vi "STPDegub.vi"(0 "object in":refnum<class "Game.lvclass">, 5 "error in (no error)":errorcluster) -> (14 "object out":refnum<class "Game.lvclass">, 19 "error out":errorcluster)   [LabVIEW 2023, in "Game.lvclass"]
uses:
  Game.lvclass
  Zone_class/zones.ctl
  Zone_class/Zone.lvclass
  Robot_class/roles.ctl
  Game.lvclass/Game.ctl
  Team_class/Team.lvclass/Team.ctl
  Field_class/Field.lvclass/Field.ctl
  PrimaryAttacker_class/PrimaryAttackerRole.lvclass
  C:/Users/ebert/Documents/codes/SSL/repo/SSL_AI/NewSTP/NewRoles/Role_v2_class/Role_v2.lvclass
  SupportAttackerRole/SupportAttackerRole.lvclass
  SupportAttackerRole/SupportAttackerRole_states.ctl
  PrimaryAttacker_class/PrimaryAttackerRole_states.ctl
  Robot_class/Robot.lvclass/Robot.ctl
  Robot_class/Write role.vi
  Read AllyRef.vi
  Read FieldRef.vi
  Field_class/Read enemyGoalPosition.vi
  Team_class/Read RobotRef.vi
  Read OffensiveTeam.vi
  Team_class/Write RobotRef.vi
  Write OffensiveTeam.vi
  Ally_class/Ally.lvclass
  C:/Users/ebert/Documents/codes/SSL/repo/SSL_AI/Team_class/Team.lvclass
  NewSTP/Playbook_v2_class/Playbook_v2.lvclass
  Field_class/Field.lvclass
  Robot_class/Robot.lvclass
  NewSTP/NewPlays/Play_v2_class/Play_v2.lvclass
  ShootTactic_v2_class/ShootTactic_v2.lvclass
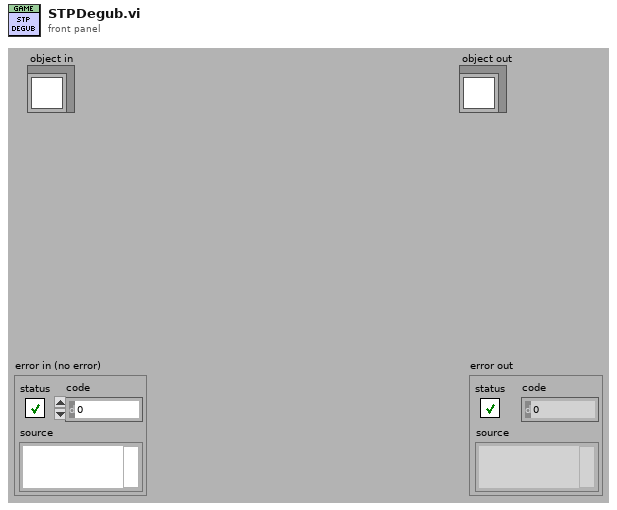
[diagram p1: front panel]
types:
  T1 = typedef "roles.ctl" = enum16{"SimpleBallPlacement", "BallPlacementAllyPasser", "BallPlacementAllyReceiver", "BallPlacementEnemy", "5Robots5th", "PassBestReceiver", "5Robots4th", "5Robots3rd", "5Robots2nd", "5Robots1st", "PassBestRobot", "WaitPass", "ABCThirdKicker", "ABCFirstKicker", "ABCSecondKicker", "Tabler", "TableFinalizer", "PrepareRollToPassRoller", "PrepareRollToPassReceiver", "SimplePassRoll", "SimplePassRollReceiver", "PenaltyDefense", "PreparePassReceiver 2", "PreparePassReceiver 1", "PassObserver", "Timeout", "Goto", "ZigZag", "None", "BallOutOfField", "DefenderArea", "Duelist", "AttackerStop", "FollowAttacker", "KeeperRole", "KickPenalty", "AttackerAimGoal", "AttackerBlock", "Marker", "Halt", "Shoot", "PassKicker", "PassReceiver", "TestRole", "PenaltyAttacker", "PrimaryAttackerRole", "SupportAttackerRole"}
  T2 = typedef "Zone.lvclass/zones.ctl" = enum16{"leftMidField", "rightMidField", "MidField", "leftWing", "rightWing", "LeftSide", "RightSide", "Field", "Size"}
  T3 = typedef "PrimaryAttackerRole.lvclass/PrimaryAttackerRole_states.ctl" = enum16{"Intercept", "PrepareShot", "Shoot", "Pass"}
  T4 = typedef "SupportAttackerRole.lvclass/SupportAttackerRole_states.ctl" = enum16{"Position", "WaitPass", "Exit"}
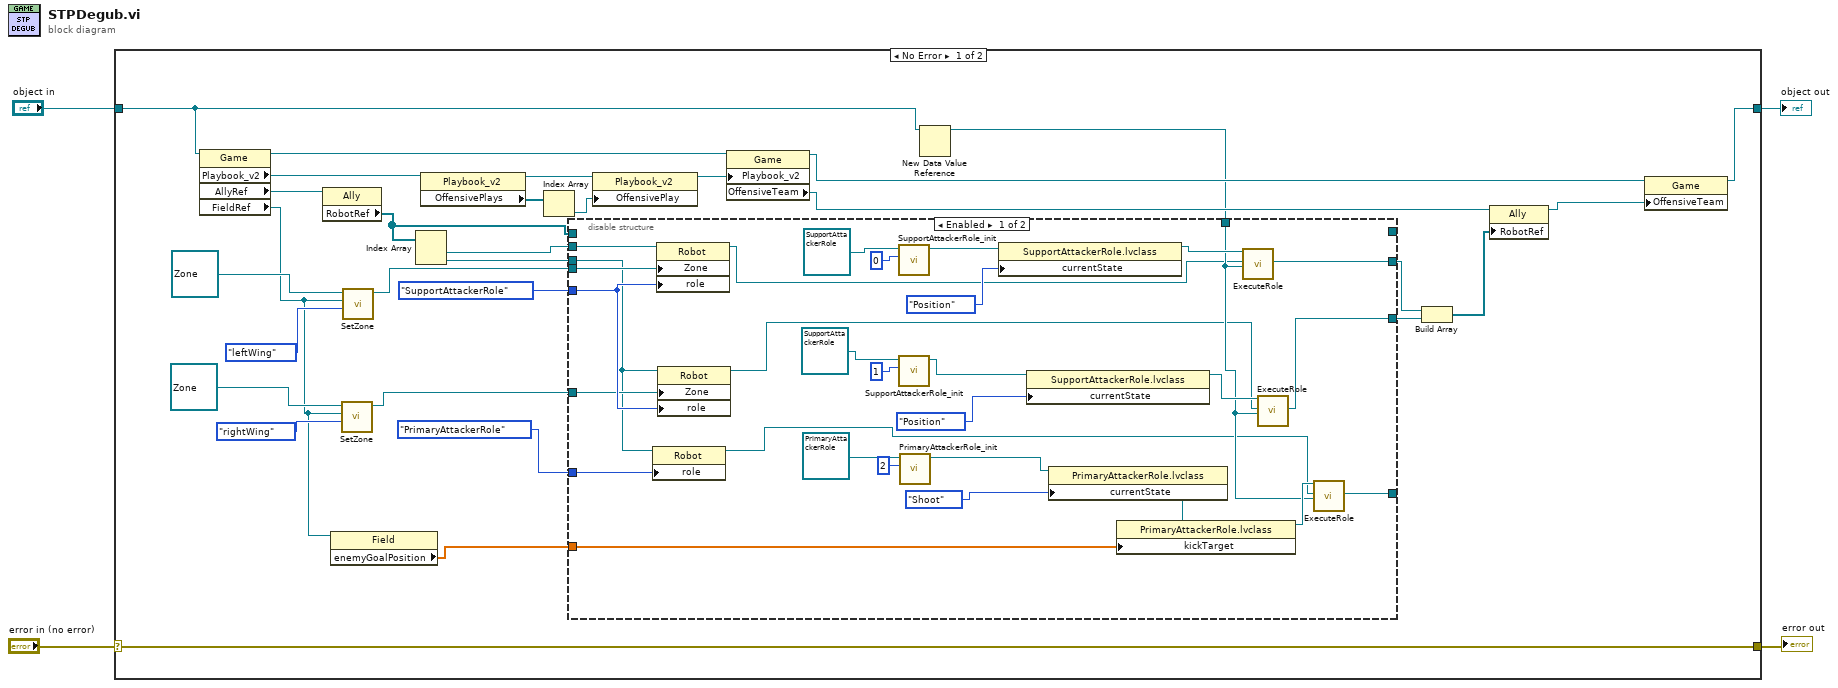
[diagram p0: block diagram]
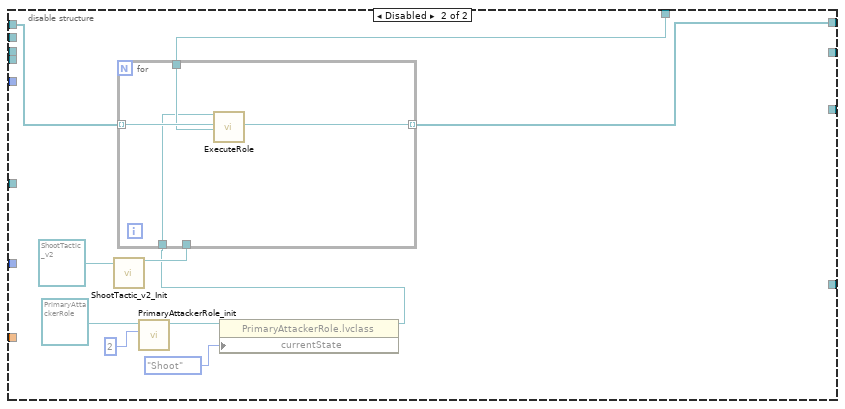
[diagram p2: hidden frame]
diagram:
  n1 = case shown="No Error" "error in (no error)" {
    selector: "error in (no error)" -> [w34 w80]
    tunnel: [w34 w80] -> w3
    tunnel: [w14 w79] -> w1
    tunnel: "object in" -> [w15 w79]
    frame No Error {
      n2 = property class="Game"(reference=w15) -> (reference out=w20:refnum<class "Game.lvclass">, "Playbook_v2"=w33:refnum<class "Playbook_v2.lvclass">, "AllyRef"=w29:refnum<class "Ally.lvclass">, "FieldRef"=w13:refnum<class "Field.lvclass">)  [unwired: 1 in, 1 out]
      n3 = property class="Ally"(reference=w29) -> ("RobotRef"=w8:refnum<class "Robot.lvclass">[])  [unwired: 1 in, 2 out]
      n4 = property class="Field"(reference=w13) -> ("enemyGoalPosition"=w12:dbl[])  [unwired: 1 in, 2 out]
      n5 = call-dynamic "SetZone.vi"("Enum"=zones."rightWing", "Field"=w13, "object in"=refnum<class "Zone.lvclass"> refnum ("Zone")) -> ("object out"=w24:refnum<class "Zone.lvclass">)  [unwired: 7 in, 1 out]
      n6 = call-dynamic "SetZone.vi"("Enum"=zones."leftWing", "Field"=w13, "object in"=refnum<class "Zone.lvclass"> refnum ("Zone")) -> ("object out"=w22:refnum<class "Zone.lvclass">)  [unwired: 7 in, 1 out]
      n7 = Index Array(array=w8) -> (element #1=w10:refnum<class "Robot.lvclass">, element #2=w9:refnum<class "Robot.lvclass">)  [unwired: 2 in]
      n8 = property class="Playbook_v2"(reference=w33) -> (reference out=w31:refnum<class "Playbook_v2.lvclass">, "OffensivePlays"=w32:refnum<class "Play_v2.lvclass">[])  [unwired: 1 in, 1 out]
      n9 = Index Array(array=w32) -> (element=w30:refnum<class "Play_v2.lvclass">)  [unwired: 1 in]
      n10 = property class="Playbook_v2"(reference=w31, "OffensivePlay"=w30) -> (reference out=w19:refnum<class "Playbook_v2.lvclass">)  [unwired: 1 in, 1 out]
      n11 = property class="Game"(reference=w20, "Playbook_v2"=w19) -> (reference out=w16:refnum<class "Game.lvclass">, "OffensiveTeam"=w17:refnum<class "Ally.lvclass">)  [unwired: 1 in, 1 out]
      n12 = New Data Value Reference(data value=w15) -> (data value reference=w11:refnum<data-value>)  [unwired: 1 in, 1 out]
      n13 = disable-structure shown="Enabled" {
        disable-tunnel: roles."SupportAttackerRole" ("role") -> [w64 _]
        disable-tunnel: w24 -> [w63 _]
        disable-tunnel: w22 -> [w62 _]
        disable-tunnel: roles."PrimaryAttackerRole" ("role") -> [w61 _]
        disable-tunnel: w12 -> [w45 _]
        disable-tunnel: w11 -> [w42 w66]
        disable-tunnel: w10 -> [w43 _]
        disable-tunnel: w9 -> [w35 _]
        disable-tunnel: [w41 _] -> _
        disable-tunnel: w8 -> [_ w74]
        disable-tunnel: [_ w65] -> _
        disable-tunnel: [w37 _] -> w7
        disable-tunnel: [w36 _] -> w6
        frame Enabled {
          n14 = property class="Robot"(reference=w35, "role"=w61) -> (reference out=w38:refnum<class "Robot.lvclass">)  [unwired: 1 in, 1 out]
          n15 = property class="Robot"(reference=w43, "Zone"=w62, "role"=w64) -> (reference out=w40:refnum<class "Robot.lvclass">)  [unwired: 1 in, 1 out]
          n16 = property class="Robot"(reference=w35, "Zone"=w63, "role"=w64) -> (reference out=w39:refnum<class "Robot.lvclass">)  [unwired: 1 in, 1 out]
          n17 = call-dynamic "SupportAttackerRole_init.vi"("roleIndex"=u8 0, "SupportAttackerRole in"=refnum<class "SupportAttackerRole.lvclass"> refnum ("SupportAttackerRole.lvclass")) -> ("SupportAttackerRole out"=w54:refnum<class "SupportAttackerRole.lvclass">)  [unwired: 8 in, 1 out]
          n18 = call-dynamic "SupportAttackerRole_init.vi"("roleIndex"=u8 1, "SupportAttackerRole in"=refnum<class "SupportAttackerRole.lvclass"> refnum ("SupportAttackerRole.lvclass")) -> ("SupportAttackerRole out"=w52:refnum<class "SupportAttackerRole.lvclass">)  [unwired: 8 in, 1 out]
          n19 = call-dynamic "PrimaryAttackerRole_init.vi"("roleIndex"=u8 2, "PrimaryAttackerRole in"=refnum<class "PrimaryAttackerRole.lvclass"> refnum ("PrimaryAttackerRole.lvclass")) -> ("PrimaryAttackerRole out"=w50:refnum<class "PrimaryAttackerRole.lvclass">)  [unwired: 8 in, 1 out]
          n20 = property class="SupportAttackerRole.lvclass"(reference=w54, "currentState"=SupportAttackerRole_states."Position" ("States")) -> (reference out=w48:refnum<class "SupportAttackerRole.lvclass">)  [unwired: 1 in, 1 out]
          n21 = property class="SupportAttackerRole.lvclass"(reference=w52, "currentState"=SupportAttackerRole_states."Position" ("States")) -> (reference out=w47:refnum<class "SupportAttackerRole.lvclass">)  [unwired: 1 in, 1 out]
          n22 = property class="PrimaryAttackerRole.lvclass"(reference=w50, "currentState"=PrimaryAttackerRole_states."Shoot" ("Enum")) -> (reference out=w46:refnum<class "PrimaryAttackerRole.lvclass">)  [unwired: 1 in, 1 out]
          n23 = property class="PrimaryAttackerRole.lvclass"(reference=w46, "kickTarget"=w45) -> (reference out=w44:refnum<class "PrimaryAttackerRole.lvclass">)  [unwired: 1 in, 1 out]
          n24 = call-dynamic "ExecuteRole.vi"("object in"=w48, "Robot in"=w40, "GameRef"=w42) -> ("Robot out"=w36:refnum<class "Robot.lvclass">)  [unwired: 14 in, 2 out]
          n25 = call-dynamic "ExecuteRole.vi"("object in"=w47, "Robot in"=w39, "GameRef"=w42) -> ("Robot out"=w37:refnum<class "Robot.lvclass">)  [unwired: 14 in, 2 out]
          n26 = call-dynamic "ExecuteRole.vi"("object in"=w44, "Robot in"=w38, "GameRef"=w42) -> ("Robot out"=w41:refnum<class "Robot.lvclass">)  [unwired: 14 in, 2 out]
        }
        frame Disabled {
          n27 = call "ShootTactic_v2_Init.vi"("object in"=refnum<class "ShootTactic_v2.lvclass"> refnum ("ShootTactic_v2")) -> ("object out"=w68:refnum<class "ShootTactic_v2.lvclass">)  [unwired: 17 in, 1 out]
          n28 = call-dynamic "PrimaryAttackerRole_init.vi"("roleIndex"=u8 2, "PrimaryAttackerRole in"=refnum<class "PrimaryAttackerRole.lvclass"> refnum ("PrimaryAttackerRole.lvclass")) -> ("PrimaryAttackerRole out"=w71:refnum<class "PrimaryAttackerRole.lvclass">)  [unwired: 8 in, 1 out]
          n29 = property class="PrimaryAttackerRole.lvclass"(reference=w71, "currentState"=PrimaryAttackerRole_states."Shoot" ("Enum")) -> (reference out=w67:refnum<class "PrimaryAttackerRole.lvclass">)  [unwired: 1 in, 1 out]
          n30 = for {
            tunnel: w74 -> [w78] mode=indexing
            tunnel: w67 -> [w76]
            tunnel: w66 -> [w77]
            tunnel: w68 -> [_]
            tunnel: [w75] -> w65 mode=indexing
            n31 = call-dynamic "ExecuteRole.vi"("object in"=w76, "Robot in"=w78, "GameRef"=w77) -> ("Robot out"=w75:refnum<class "Robot.lvclass">)  [unwired: 14 in, 2 out]
          }
        }
      }
      n32 = Build Array(w6, w7) -> (w5:refnum<class "Robot.lvclass">[])
      n33 = property class="Ally"(reference=w17, "RobotRef"=w5) -> (reference out=w18:refnum<class "Ally.lvclass">)  [unwired: 1 in, 1 out]
      n34 = property class="Game"(reference=w16, "OffensiveTeam"=w18) -> (reference out=w14:refnum<class "Game.lvclass">)  [unwired: 1 in, 1 out]
    }
    frame Error {
    }
  }
  "error out" <- w3
  "object out" <- w1
